vi "M05 Hydraulic cells v2.vi"(11 "EV3 in":T1) -> (3 "EV3 out":T1)   [LabVIEW 2016]
uses:
  <vilib>/NXT/Subs/LVHSConnector.ctl
  <vilib>/NXT/LegoClasses/BrickReference/BrickReference.lvclass
  <vilib>/NXT/Dual Mode Library/Waits/Wait_Num.vi
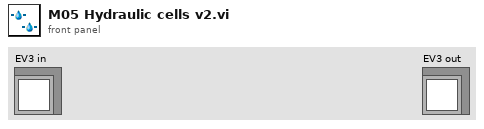
[diagram p1: front panel]
types:
  T1 = typedef "LVHSConnector.ctl" = refnum<class "BrickReference.lvclass">
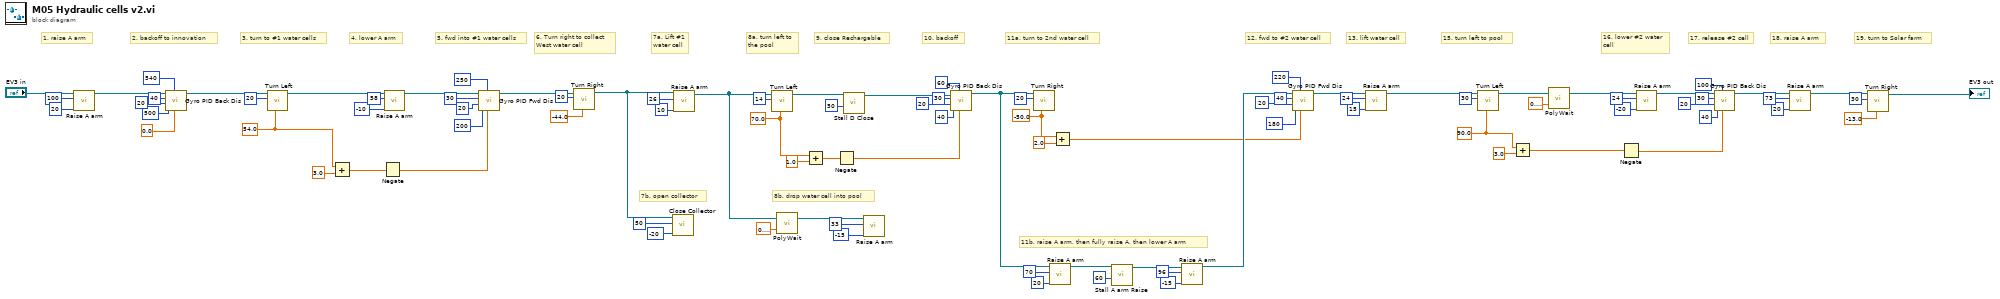
[diagram p0: block diagram]
diagram:
  w14 = sgl 90.0 ("Turning angle")
  w44 = sgl -50.0 ("Turning angle")
  w47 = sgl 70.0 ("Turning angle")
  w72 = sgl 54.0 ("Turning angle")
  # "19. turn to Solar farm"
  # "18. raise A arm"
  # "17. release #2 cell"
  # "16. lower #2 water\ncell"
  # "15. turn left to pool"
  # "13. lift water cell"
  # "9. close Rechargable"
  # "7b. open collector"
  # "12. fwd to #2 water cell"
  # "11b. raise A arm, then fully raise A, then lower A arm"
  # "11a. turn to 2nd water cell"
  # "10. backoff"
  # "8b. drop water cell into pool"
  # "8a. turn left to\nthe pool"
  # "7a. Lift #1\nwater cell"
  # "6. Turn right to collect\nWest water cell"
  # "5. fwd into #1 water cells"
  # "4. lower A arm"
  # "3. turn to #1 water cells"
  # "2. backoff to innovation"
  # "1. raise A arm"
  n1 = call "Raise A arm.vi"("Power"=i8 20, "Rotation"=100, "EV3 in"="EV3 in") -> ("EV3 out"=w88:T1)  [unwired: 8 in]
  n2 = call "Gyro PID Back Dis.vi"("Target angle"=sgl 0.0, "Threshold to stop"=540 ("Threshold to Color"), "Threshold to slow"=500, "Min. speed"=20, "Max. speed"=40, "EV3 in"=w88) -> ("EV3 out"=w82:T1)  [unwired: 5 in]
  n3 = call "Turn Left.vi"("Turning angle"=w72, "Motor B (right)"=i8 20, "EV3 in"=w82) -> ("EV3 out"=w75:T1)  [unwired: 8 in]
  n4 = Add(x=w72, y=sgl 3.0) -> (x+y=w70:sgl)
  n5 = Negate(x=w70) -> (-x=w69:sgl)
  n6 = call "Raise A arm.vi"("Power"=i8 -10, "Rotation"=58, "EV3 in"=w75) -> ("EV3 out"=w73:T1)  [unwired: 8 in]
  n7 = call "Gyro PID Fwd Dis.vi"("Target angle"=w69, "Threshold to stop"=250, "Threshold to slow"=200, "Min. speed"=20, "Max. speed"=30, "EV3 in"=w73) -> ("EV3 out"=w68:T1)  [unwired: 5 in]
  n8 = call "Turn Right.vi"("Turning angle"=sgl -44.0, "Motor B (right)"=i8 20, "EV3 in"=w68) -> ("EV3 out"=w40:T1)  [unwired: 8 in]
  n9 = call "Close Collector.vi"("Power"=i8 -20, "Rotation"=50, "EV3 in"=w40) -> ()  [unwired: 8 in, 1 out]
  n10 = call "Raise A arm.vi"("Power"=i8 10, "Rotation"=26, "EV3 in"=w40) -> ("EV3 out"=w38:T1)  [unwired: 8 in]
  n11 = call "Turn Left.vi"("Turning angle"=w47, "Motor B (right)"=i8 14, "EV3 in"=w38) -> ("EV3 out"=w37:T1)  [unwired: 8 in]
  n12 = call-poly <vilib>:"PolyWait.vi"("Time (1 sec)"=sgl 0.6, "NXT/EV3"=w38) -> ("NXT/EV3"=w43:T1)  [unwired: 2 in]
  n13 = Add(x=w47, y=sgl 1.0) -> (x+y=w46:sgl)
  n14 = Negate(x=w46) -> (-x=w35:sgl)
  n15 = call "Stall D Close.vi"("Power"=i8 50, "NXT/EV3"=w37) -> ("NXT/EV3"=w36:T1)  [unwired: 9 in]
  n16 = call "Raise A arm.vi"("Power"=i8 -15, "Rotation"=33, "EV3 in"=w43) -> ()  [unwired: 8 in, 1 out]
  n17 = call "Gyro PID Back Dis.vi"("Target angle"=w35, "Threshold to stop"=60, "Threshold to slow"=40, "Min. speed"=20, "Max. speed"=30, "EV3 in"=w36) -> ("EV3 out"=w49:T1)  [unwired: 5 in]
  n18 = call "Turn Right.vi"("Turning angle"=w44, "Motor B (right)"=i8 20, "EV3 in"=w49) -> ()  [unwired: 8 in, 1 out]
  n19 = call "Raise A arm.vi"("Power"=i8 20, "Rotation"=70, "EV3 in"=w49) -> ("EV3 out"=w33:T1)  [unwired: 8 in]
  n20 = Add(x=w44, y=sgl 2.0) -> (x+y=w24:sgl)
  n21 = call "Stall A arm Raise.vi"("Power"=i8 60, "NXT/EV3"=w33) -> ("NXT/EV3"=w29:T1)  [unwired: 9 in]
  n22 = call "Raise A arm.vi"("Power"=i8 -15, "Rotation"=96, "EV3 in"=w29) -> ("EV3 out"=w28:T1)  [unwired: 8 in]
  n23 = call "Gyro PID Fwd Dis.vi"("Target angle"=w24, "Threshold to stop"=220, "Threshold to slow"=180, "Min. speed"=20, "Max. speed"=40, "EV3 in"=w28) -> ("EV3 out"=w25:T1)  [unwired: 5 in]
  n24 = call "Raise A arm.vi"("Power"=i8 15, "Rotation"=24, "EV3 in"=w25) -> ("EV3 out"=w1:T1)  [unwired: 8 in]
  n25 = call "Turn Left.vi"("Turning angle"=w14, "Motor B (right)"=i8 30, "EV3 in"=w1) -> ("EV3 out"=w21:T1)  [unwired: 8 in]
  n26 = Add(x=w14, y=sgl 3.0) -> (x+y=w13:sgl)
  n27 = call-poly <vilib>:"PolyWait.vi"("Time (1 sec)"=sgl 0.4, "NXT/EV3"=w21) -> ("NXT/EV3"=w3:T1)  [unwired: 2 in]
  n28 = Negate(x=w13) -> (-x=w12:sgl)
  n29 = call "Raise A arm.vi"("Power"=i8 -20, "Rotation"=24, "EV3 in"=w3) -> ("EV3 out"=w16:T1)  [unwired: 8 in]
  n30 = call "Gyro PID Back Dis.vi"("Target angle"=w12, "Threshold to stop"=100, "Threshold to slow"=40, "Min. speed"=20, "Max. speed"=30, "EV3 in"=w16) -> ("EV3 out"=w5:T1)  [unwired: 5 in]
  n31 = call "Raise A arm.vi"("Power"=i8 20, "Rotation"=73, "EV3 in"=w5) -> ("EV3 out"=w4:T1)  [unwired: 8 in]
  n32 = call "Turn Right.vi"("Turning angle"=sgl -13.0, "Motor B (right)"=i8 30, "EV3 in"=w4) -> ("EV3 out"=→"EV3 out":T1)  [unwired: 8 in]
